vi "Convert 2D mask to 2D array mask.vi"(11 "image data":T1) -> (3 "2D Mask":u8[][](array[numeric]))   [LabVIEW 2019]
uses:
  <vilib>/picture/picture.llb/imagedata.ctl
panel:
  out "Init Data Out":u8[](array[numeric])
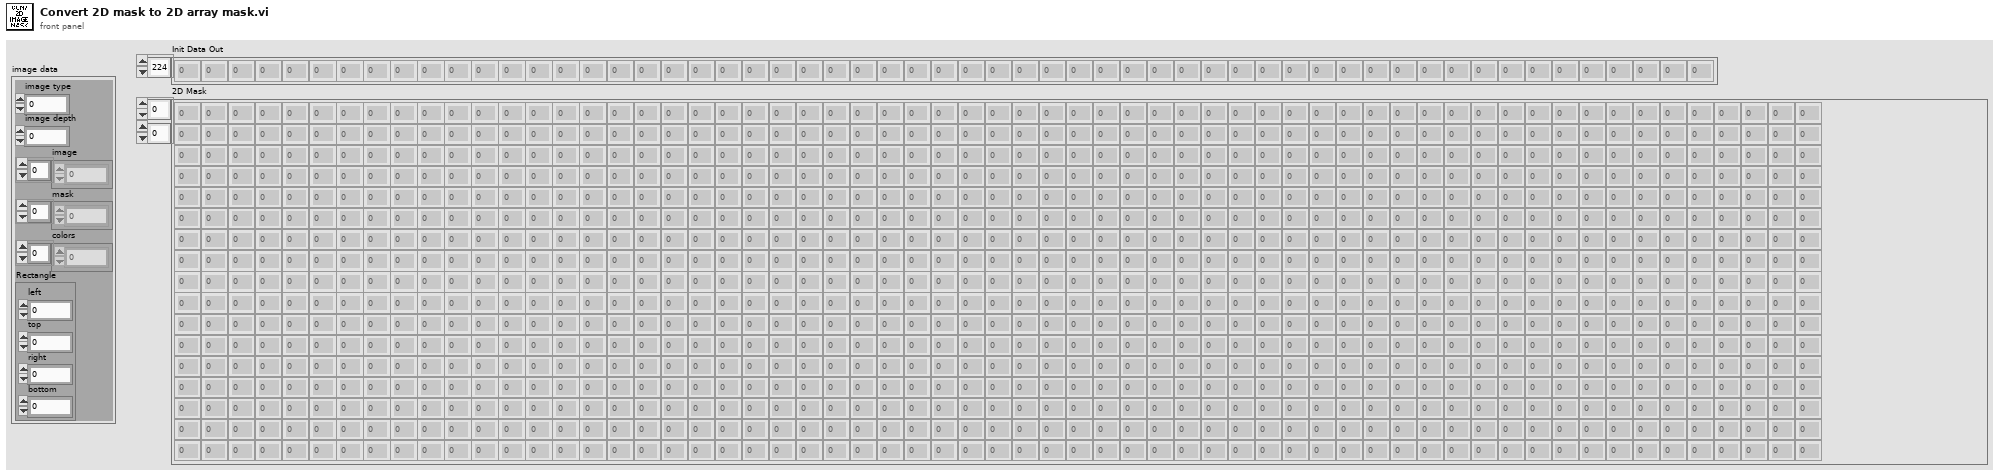
[diagram p1: front panel]
types:
  T1 = typedef "imagedata.ctl" = cluster{"image type":i32, "image depth":i32, "image":u8[], "mask":u8[], "colors":u32[], "Rectangle":cluster{"left":i16, "top":i16, "right":i16, "bottom":i16}}
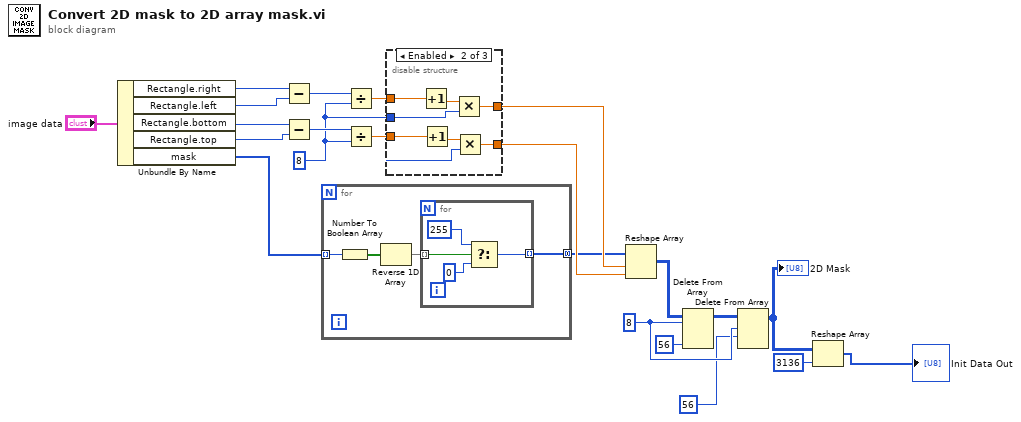
[diagram p0: block diagram]
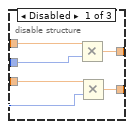
[diagram p2: hidden frame]
diagram:
  w5 = 8 ("length")
  w16 = i16 8 ("x")
  n1 = Unbundle By Name("image data") -> ("Rectangle.right"=w9:i16, "Rectangle.left"=w17:i16, "Rectangle.bottom"=w10:i16, "Rectangle.top"=w18:i16, "mask"=w21:u8[])
  n2 = Subtract(x=w9, y=w17) -> (x-y=w20:i16)
  n3 = Subtract(x=w10, y=w18) -> (x-y=w19:i16)
  n4 = for {
    tunnel: w21 -> [w26] mode=indexing
    tunnel: [w23] -> w11 mode=concatenating
    n5 = Number To Boolean Array(number=w26) -> (Boolean array=w25:bool[])
    n6 = Reverse 1D Array(array=w25) -> (reversed array=w24:bool[])
    n7 = for {
      tunnel: w24 -> [w30] mode=indexing
      tunnel: [w27] -> w23 mode=indexing
      n8 = Select(t=u8 255, s=w30, f=u8 0) -> (s? t:f=w27:u8)
    }
  }
  n9 = Divide(x=w20, y=w16) -> (x/y=w12:dbl)
  n10 = Divide(x=w19, y=w16) -> (x/y=w14:dbl)
  n11 = disable-structure shown="Enabled" {
    disable-tunnel: w16 -> [w35 w42 _]
    disable-tunnel: [w34 w41 _] -> w15
    disable-tunnel: w14 -> [w33 w40 _]
    disable-tunnel: [w32 w38 _] -> w13
    disable-tunnel: w12 -> [w31 w36 _]
    frame Disabled {
      n12 = Multiply(x=w31, y=w35) -> (x*y=w32:dbl)
      n13 = Multiply(x=w33, y=w35) -> (x*y=w34:dbl)
    }
    frame Enabled {
      n14 = Increment(x=w36) -> (x+1=w37:dbl)
      n15 = Increment(x=w40) -> (x+1=w39:dbl)
      n16 = Multiply(x=w37, y=w42) -> (x*y=w38:dbl)
      n17 = Multiply(x=w39, y=w42) -> (x*y=w41:dbl)
    }
    frame Disabled {
    }
  }
  n18 = Reshape Array(w11, w13, w15) -> (w8:u8[][])
  n19 = Delete From Array(array=w8, length=w5, index (col)=56 ("disabled index (col)")) -> (array with subset deleted=w6:u8[][])  [unwired: 1 in, 1 out]
  n20 = Delete From Array(array=w6, length=w5, index (row)=56) -> (array with subset deleted=w3:u8[][])  [unwired: 1 in, 1 out]
  "2D Mask" <- w3
  n21 = Reshape Array(w3, 3136 ("dimension size")) -> (→"Init Data Out":u8[])
